vi "hidSPD List Devices.vi"(8 "error in (no error)":errorcluster) -> (0 "error out":errorcluster, 2 "List":string[][](array[string]))   [LabVIEW 2018, in "hidSPDLibForLabView.lvlib"]
uses:
  hidSPDLibForLabView.lvlib
  hidSPD DLL files/libSPD.dll
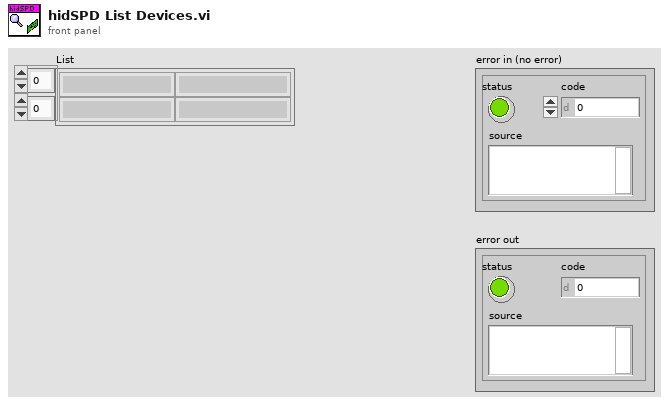
[diagram p1: front panel]
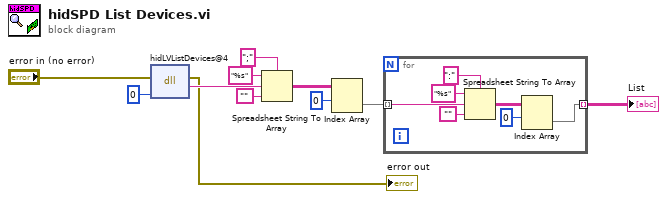
[diagram p0: block diagram]
diagram:
  n1 = dll-call lib="F:/NextCloud/SPD stand/hidSPDLibForLabView/hidSPD DLL files/libSPD.dll" fn="hidLVListDevices@4"(error in="error in (no error)", "listLength"=0) -> (error out=→"error out":errorcluster, "return type"=w9:string)  [unwired: 3 in, 1 out]
  n2 = Spreadsheet String To Array(delimiter (Tab)=";", format string="%s", spreadsheet string=w9, array type (2D Dbl)="") -> (array=w4:string[][])
  n3 = Index Array(array=w4, index (row)=0) -> (element=w2:string[])  [unwired: 1 in]
  n4 = for {
    tunnel: w2 -> [w15] mode=indexing
    tunnel: [w14] -> w1 mode=indexing
    n5 = Spreadsheet String To Array(delimiter (Tab)=":", format string="%s", spreadsheet string=w15, array type (2D Dbl)="") -> (array=w13:string[][])
    n6 = Index Array(array=w13, index (row)=0) -> (element=w14:string[])  [unwired: 1 in]
  }
  "List" <- w1
